vi "demo - pico adc continuous.vi"() -> ()   [LabVIEW 2024]
doc: "#vi_description \nPlot a ADC data onto a waveform chart until the user presses stop or an error has occurred.\nThetic Engineering Ltd."
uses:
  <instrlib>/HandsOnPi2040/Public/AnaIns.ctl
  <instrlib>/HandsOnPi2040/HandsOnPi2040.lvlib
panel:
  in  "Stop":bool
  out "Waveform Chart":u16(graph)
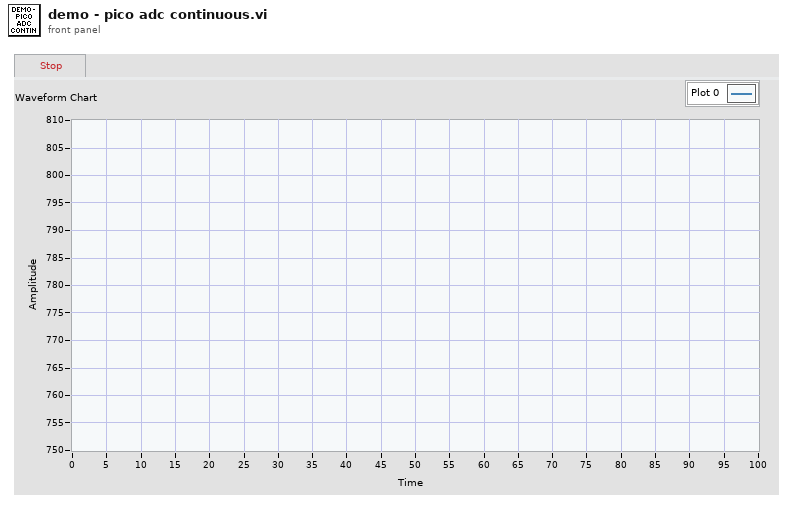
[diagram p1: front panel]
types:
  T1 = typedef "HandsOnPi2040.lvlib/AnaIns.ctl" = enum16{"No AI - Error", "AI1", "AI2"}
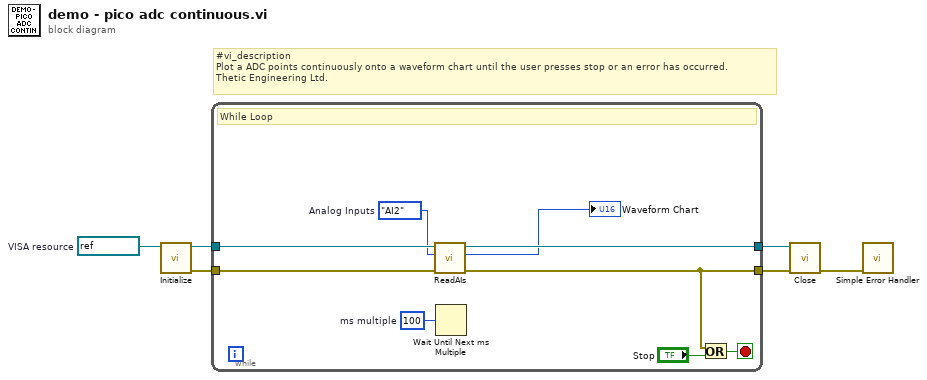
[diagram p0: block diagram]
diagram:
  w2 = refnum<visa-resource-name> "COM3"  # VISA resource
  # "#vi_description \nPlot a ADC points continuously onto a waveform chart until the user presses stop or an error has occurred.\nThetic Engineering Ltd."
  n1 = call <instrlib>:"Initialize.vi"("VISA resource name"=w2) -> ("error out"=w5:errorcluster, "VISA resource name out"=w6:refnum<visa-resource-name>)  [unwired: 8 in, 1 out]
  n2 = while {
    tunnel: w6 -> [w13]
    tunnel: w5 -> [w12]
    tunnel: [w11] -> w4
    tunnel: [w7] -> w3
    stop <- w8 stop-if-true
    w10 = AnaIns."AI2"  # Analog Inputs
    w14 = u32 100  # ms multiple
    # "While Loop"
    n3 = call <instrlib>:"ReadAIs.vi"("error in (no error)"=w12, "Analog Inputs"=w10, "VISA resource name"=w13) -> ("error out"=w7:errorcluster, "Value"=→"Waveform Chart":u16, "VISA resource name out"=w11:refnum<visa-resource-name>)  [unwired: 6 in]
    n4 = Wait Until Next ms Multiple(millisecond multiple=w14) -> ()  [unwired: 1 out]
    n5 = Or(x=w7, y="Stop") -> (x .or. y?=w8:bool)
  }
  n6 = call <instrlib>:"Close.vi"("error in (no error)"=w3, "VISA resource name"=w4) -> ("error out"=w1:errorcluster)  [unwired: 9 in]
  n7 = call <vilib>:"Simple Error Handler.vi"("error in (no error)"=w1) -> ()  [unwired: 4 in, 5 out]
